vi "Create Data Channels.vi"(8 "error in":errorcluster, 11 "Node in":refnum<class "ThermotronDriver.lvclass">) -> (0 "error out":errorcluster, 3 "Node out":refnum<class "ThermotronDriver.lvclass">)   [LabVIEW 2023, in "ThermotronDriver.lvlib" / "ThermotronDriver.lvclass"]
uses:
  ThermotronDriver.lvclass
  ThermotronDriver.lvclass/ThermotronDriver.ctl
  <vilib>/ADAS Replay HIL/Channels/Tag Wrapper/Tag Wrapper.lvlib
  <vilib>/ADAS Replay HIL/Channels/Tag Wrapper/Polymorphic/Open Producer Tag (Double).vi
  <vilib>/ADAS Replay HIL/Template Node/Plugin/Template Node/Template Node.lvclass
  <vilib>/ADAS Replay HIL/Template Node/Plugin/Template Node/Data Channel/Get Tag Producer Channel Name.vi
  <vilib>/ADAS Replay HIL/Channels/Tag Wrapper/Polymorphic/Write Channel (Double).vi
  <vilib>/ADAS Replay HIL/Channels/Tag Wrapper/Polymorphic/Open Consumer Tag (Double).vi
  <vilib>/ADAS Replay HIL/Template Node/Plugin/Template Node/Data Channel/Get Tag Consumer Channel Name.vi
  <vilib>/ADAS Replay HIL/Channels/Tag Wrapper/Polymorphic/Set Default Value (Double).vi
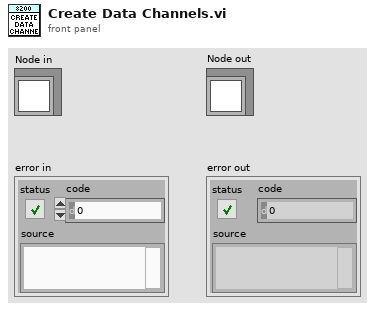
[diagram p1: front panel]
types:
  T1 = typedef "Template Node.lvlib/Template Node.lvclass/Data Channel Info.ctl" = cluster{"Channel Name":string, "Type Description":string}
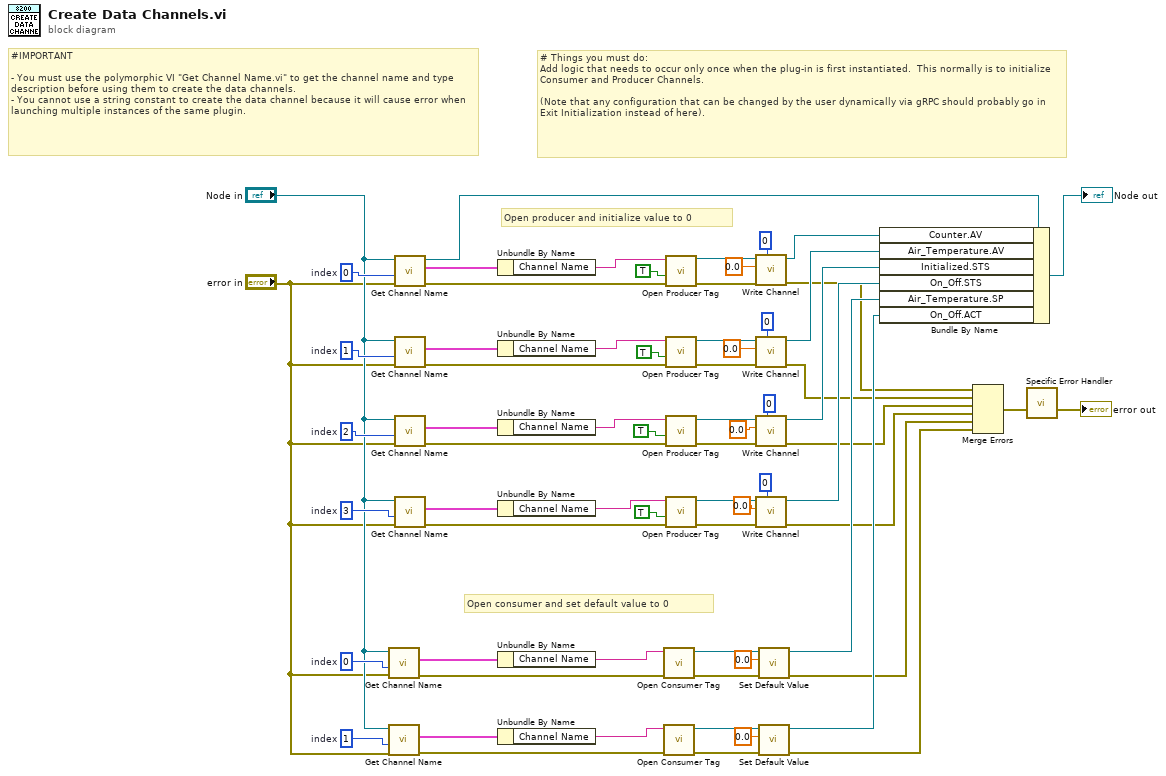
[diagram p0: block diagram]
diagram:
  w14 = 1  # index
  w25 = 0  # index
  w57 = 3  # index
  w52 = 2  # index
  w58 = 1  # index
  w66 = 0  # index
  # "Open consumer and set default value to 0"
  # "Open producer and initialize value to 0"
  # "# Things you must do:\nAdd logic that needs to occur only once when the plug-in is first instantiated.  This normally is to initialize Consumer and Producer Channels.   \n\n(Note that any configuration that can be changed by the user dynamically via gRPC should probably go in Exit Initialization instead of here)."
  # "#IMPORTANT\n\n- You must use the polymorphic VI \"Get Channel Name.vi\" to get the channel name and type description before using them to create the data channels.\n- You cannot use a string constant to create the data channel because it will cause error when launching multiple instances of the same plugin."
  n1 = call-poly <vilib>:"Get Channel Name.vi"("error in"="error in", "index"=w25, "Node in"="Node in") -> ("error out"=w22:errorcluster, "Channel Name"=w24:T1)  [unwired: 6 in, 1 out]
  n2 = call-poly <vilib>:"Get Channel Name.vi"("error in"="error in", "index"=w14, "Node in"="Node in") -> ("error out"=w17:errorcluster, "Channel Name"=w15:T1)  [unwired: 6 in, 1 out]
  n3 = call-poly <vilib>:"Get Channel Name.vi"("error in"="error in", "index"=w66, "Node in"="Node in") -> ("error out"=w62:errorcluster, "Channel Name"=w65:T1, "Node out"=w67:refnum<class "ThermotronDriver.lvclass">)  [unwired: 6 in]
  n4 = call-poly <vilib>:"Get Channel Name.vi"("error in"="error in", "index"=w58, "Node in"="Node in") -> ("error out"=w59:errorcluster, "Channel Name"=w46:T1)  [unwired: 6 in, 1 out]
  n5 = call-poly <vilib>:"Get Channel Name.vi"("error in"="error in", "index"=w52, "Node in"="Node in") -> ("error out"=w53:errorcluster, "Channel Name"=w47:T1)  [unwired: 6 in, 1 out]
  n6 = call-poly <vilib>:"Get Channel Name.vi"("error in"="error in", "index"=w57, "Node in"="Node in") -> ("error out"=w56:errorcluster, "Channel Name"=w48:T1)  [unwired: 6 in, 1 out]
  n7 = Unbundle By Name(w65) -> ("Channel Name"=w63:string)
  n8 = Unbundle By Name(w46) -> ("Channel Name"=w51:string)
  n9 = Unbundle By Name(w47) -> ("Channel Name"=w50:string)
  n10 = Unbundle By Name(w48) -> ("Channel Name"=w49:string)
  n11 = Unbundle By Name(w24) -> ("Channel Name"=w23:string)
  n12 = Unbundle By Name(w15) -> ("Channel Name"=w16:string)
  n13 = call-poly <vilib>:"Open Consumer Tag.vi"("error in"=w22, "Channel Name"=w23) -> ("error out"=w20:errorcluster, "ADAS HIL Channel"=w21:refnum<k21>)  [unwired: 8 in]
  n14 = call-poly <vilib>:"Open Consumer Tag.vi"("error in"=w17, "Channel Name"=w16) -> ("error out"=w19:errorcluster, "ADAS HIL Channel"=w18:refnum<k21>)  [unwired: 8 in]
  n15 = call-poly <vilib>:"Open Producer Tag.vi"("error in"=w62, "Create if not found? (T)"=TRUE, "Channel Name"=w63) -> ("error out"=w43:errorcluster, "ADAS HIL Channel"=w45:refnum<k21>)  [unwired: 7 in]
  n16 = call-poly <vilib>:"Open Producer Tag.vi"("error in"=w59, "Create if not found? (T)"=TRUE, "Channel Name"=w51) -> ("error out"=w32:errorcluster, "ADAS HIL Channel"=w33:refnum<k21>)  [unwired: 7 in]
  n17 = call-poly <vilib>:"Open Producer Tag.vi"("error in"=w53, "Create if not found? (T)"=TRUE, "Channel Name"=w50) -> ("error out"=w31:errorcluster, "ADAS HIL Channel"=w34:refnum<k21>)  [unwired: 7 in]
  n18 = call-poly <vilib>:"Open Producer Tag.vi"("error in"=w56, "Create if not found? (T)"=TRUE, "Channel Name"=w49) -> ("error out"=w26:errorcluster, "ADAS HIL Channel"=w35:refnum<k21>)  [unwired: 7 in]
  n19 = call-poly <vilib>:"Write Channel.vi"("Timeout (ms)"=0, "error in"=w43, "Value to Write"=0.0, "ADAS HIL Channel in"=w45) -> ("error out"=w7:errorcluster, "ADAS HIL Channel out"=w30:refnum<k21>)  [unwired: 5 in, 1 out]
  n20 = call-poly <vilib>:"Write Channel.vi"("Timeout (ms)"=0, "error in"=w32, "Value to Write"=0.0, "ADAS HIL Channel in"=w33) -> ("error out"=w6:errorcluster, "ADAS HIL Channel out"=w29:refnum<k21>)  [unwired: 5 in, 1 out]
  n21 = call-poly <vilib>:"Write Channel.vi"("Timeout (ms)"=0, "error in"=w31, "Value to Write"=0.0, "ADAS HIL Channel in"=w34) -> ("error out"=w5:errorcluster, "ADAS HIL Channel out"=w28:refnum<k21>)  [unwired: 5 in, 1 out]
  n22 = call-poly <vilib>:"Write Channel.vi"("Timeout (ms)"=0, "error in"=w26, "Value to Write"=0.0, "ADAS HIL Channel in"=w35) -> ("error out"=w4:errorcluster, "ADAS HIL Channel out"=w27:refnum<k21>)  [unwired: 5 in, 1 out]
  n23 = call-poly <vilib>:"Set Default Value.vi"("error in"=w20, "Default Value"=0.0, "ADAS HIL Channel in"=w21) -> ("error out"=w3:errorcluster, "ADAS HIL Channel out"=w9:refnum<k21>)  [unwired: 7 in]
  n24 = call-poly <vilib>:"Set Default Value.vi"("error in"=w19, "Default Value"=0.0, "ADAS HIL Channel in"=w18) -> ("error out"=w2:errorcluster, "ADAS HIL Channel out"=w8:refnum<k21>)  [unwired: 7 in]
  n25 = Bundle By Name(cluster=w67, "Counter.AV"=w30, "Air_Temperature.AV"=w29, "Initialized.STS"=w28, "On_Off.STS"=w27, "Air_Temperature.SP"=w9, "On_Off.ACT"=w8) -> (→"Node out":refnum<class "ThermotronDriver.lvclass">)
  n26 = Merge Errors(w7, w6, w5, w4, w3, w2) -> (w1:errorcluster)
  n27 = call "Specific Error Handler"("Error to Check"=w1) -> ("error out"=→"error out":errorcluster)  [unwired: 11 in, 3 out]
